vi "SIM900 Module Comm.vi"(7 "Wait (ms)":u32=30, 8 "Error In":errorcluster, 9 "Query":string, 10 "Slot":T1(ring), 11 "VISA Resource Name":refnum<visa-resource-name>="GPIB0::3::INSTR") -> (0 "Error Out":errorcluster {"code" format="%.0x"}, 2 "Response":string, 3 "dup VISA Session":refnum<visa-resource-name>)   [LabVIEW 2019]
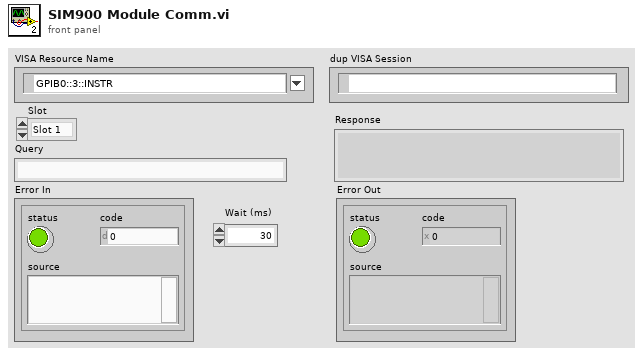
[diagram p1: front panel]
types:
  T1 = enum32{"Slot 1", "Slot 2", "Slot 3", "Slot 4", "Slot 5", "Slot 6", "Slot 7", "Slot 8"}
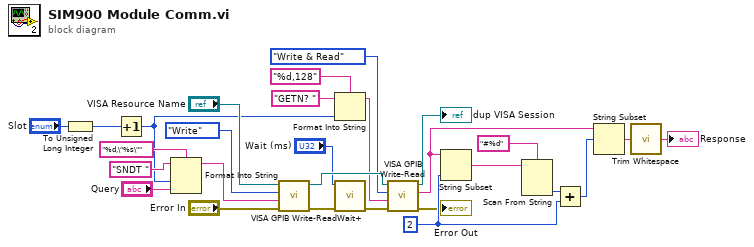
[diagram p0: block diagram]
diagram:
  w16 = 2 ("length (rest)")
  n1 = To Unsigned Long Integer(number="Slot") -> (unsigned 32bit integer=w2:u32)
  n2 = Increment(x=w2) -> (x+1=w1:u32)
  n3 = Format Into String(format string="%d,\"%s\"", initial string="SNDT ", w1, "Query") -> (resulting string=w23:string)  [unwired: 1 in, 1 out]
  n4 = call "VISA GPIB Write-Read.vi"("error in (no error)"="Error In", "Command"=w23, "Action"=enum16{"Write", "Read", "Write & Read"}."Write", "VISA resource name"="VISA Resource Name") -> ("error out"=w9:errorcluster, "dup VISA Session"=w14:refnum<visa-resource-name>)  [unwired: 4 in, 2 out]
  n5 = Format Into String(format string="%d,128", initial string="GETN? ", w1) -> (resulting string=w5:string)  [unwired: 1 in, 1 out]
  n6 = call "Wait+.vi"("Error In"=w9, "milliseconds to wait"="Wait (ms)") -> ("Error Out"=w4:errorcluster)  [unwired: 4 in, 1 out]
  n7 = call "VISA GPIB Write-Read.vi"("error in (no error)"=w4, "Command"=w5, "Action"=enum16{"Write", "Read", "Write & Read"}."Write & Read", "VISA resource name"=w14) -> ("error out"=→"Error Out":errorcluster, "String Returned"=w11:string, "dup VISA Session"=→"dup VISA Session":refnum<visa-resource-name>)  [unwired: 4 in, 1 out]
  n8 = String Subset(string=w11, length (rest)=w16) -> (substring=w20:string)  [unwired: 1 in]
  n9 = Scan From String(format string="#%d", input string=w20) -> (output 1=w18:i32)  [unwired: 3 in, 3 out]
  n10 = Add(x=w18, y=w16) -> (x+y=w17:i32)
  n11 = String Subset(string=w11, offset (0)=w17) -> (substring=w21:string)  [unwired: 1 in]
  n12 = call <vilib>:"Trim Whitespace.vi"("string"=w21) -> ("trimmed string"=→"Response":string)  [unwired: 1 in]
